vi "ShowStations.vi"(9 "Visible names?":bool=TRUE, 11 "Map":refnum<vi>) -> (3 "Map out":refnum<vi>)   [LabVIEW 2014]
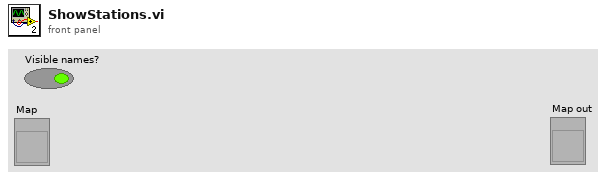
[diagram p1: front panel]
types:
  T1 = typedef "LVCursorListTypeDef.ctl" = cluster{"Name":string, "Color":u32, "Style":u8, "Point Style":u8, "Name Visible":bool, "Allow Drag":bool, "Cursor Mode":u32, "Plot":i32, "Index":i32, "Position":cluster{"X":dbl, "Y":dbl}, "X Scale":u32, "Y Scale":u32, "Watch Plots":i32[], "Watch All Plots":bool, "Plot Area":i32, "Label Offset":cluster{"X":dbl, "Y":dbl}}[]
  T2 = cluster{"Name":string, "Color":u32, "Style":u8, "Point Style":u8, "Name Visible":bool, "Allow Drag":bool, "Cursor Mode":u32, "Plot":i32, "Index":i32, "Position":cluster{"X":dbl, "Y":dbl}, "X Scale":u32, "Y Scale":u32, "Watch Plots":i32[], "Watch All Plots":bool, "Plot Area":i32, "Label Offset":cluster{"X":dbl, "Y":dbl}}
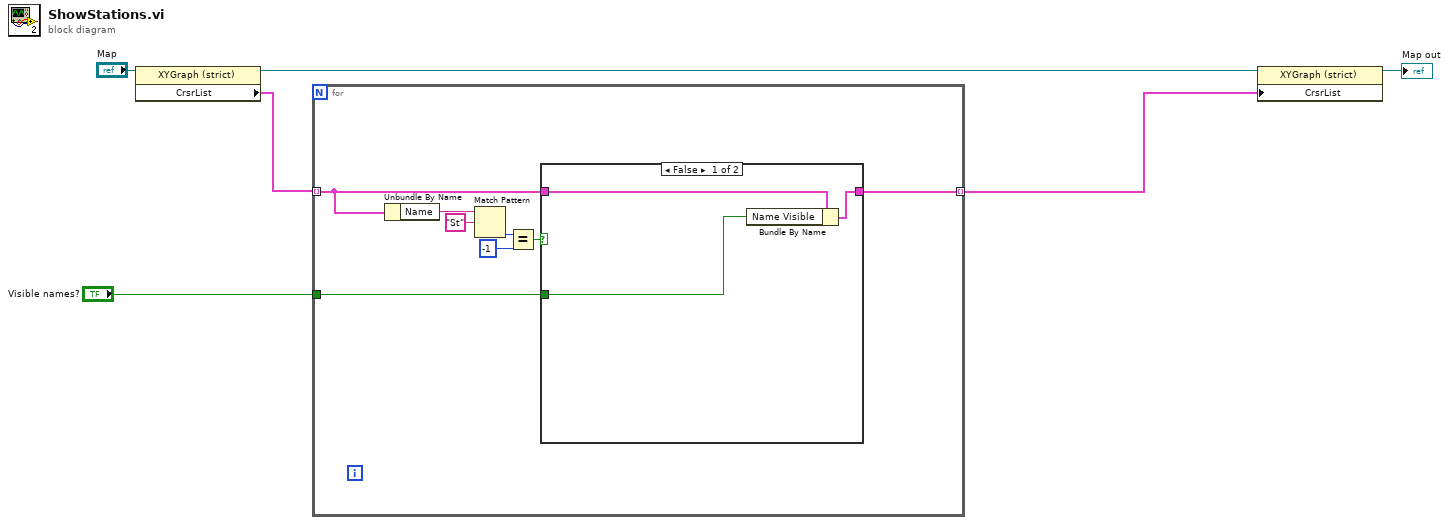
[diagram p0: block diagram]
diagram:
  n1 = property on="Property Node" class="XYGraph (strict)"(reference="Map") -> (reference out=w4:refnum<vi>, "CrsrList"=w2:T1)  [unwired: 1 in, 1 out]
  n2 = for {
    tunnel: "Visible names?" -> [w8]
    tunnel: w2 -> [w9] mode=indexing
    tunnel: [w7] -> w1 mode=indexing
    n3 = Unbundle By Name(w9) -> ("Name"=w10:string)
    n4 = Match Pattern(string=w10, regular expression="St") -> (offset past match=w12:i32)  [unwired: 1 in, 3 out]
    n5 = Equal?(x=w12, y=-1) -> (x = y?=w14:bool)
    n6 = case shown="False" w14 {
      tunnel: w9 -> [w16 w18]
      tunnel: [w17 w18] -> w7
      tunnel: w8 -> [w15 _]
      frame False {
        n7 = Bundle By Name(cluster=w16, "Name Visible"=w15) -> (w17:T2)
      }
      frame True {
      }
    }
  }
  n8 = property on="Property Node" class="XYGraph (strict)"(reference=w4, "CrsrList"=w1) -> (reference out=→"Map out":refnum<vi>)  [unwired: 1 in, 1 out]
